vi "Write DetailedResult.vi"(8 "error in (no error)":errorcluster, 10 "DetailedResult":T1, 11 "LocalReport in":refnum<class "LocalReport.lvclass">) -> (0 "error out":errorcluster, 3 "LocalReport out":refnum<class "LocalReport.lvclass">)   [LabVIEW 2019, in "LocalReport.lvlib" / "LocalReport.lvclass"]
uses:
  LocalReport.lvclass
  LocalReport.lvclass/LocalReport.ctl
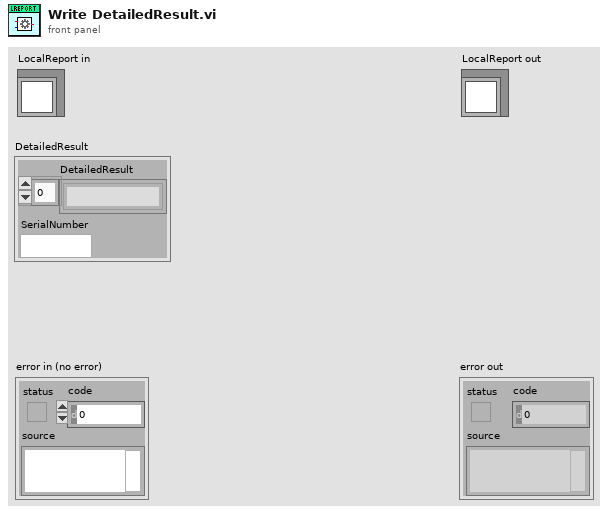
[diagram p1: front panel]
types:
  T1 = cluster{"DetailedResult":string[], "SerialNumber":string}
  T2 = cluster{"TestResultData":string[][], "SerialNumber":string}
  T3 = cluster{"TestResultData":string[][], "SerialNumber":string}[]
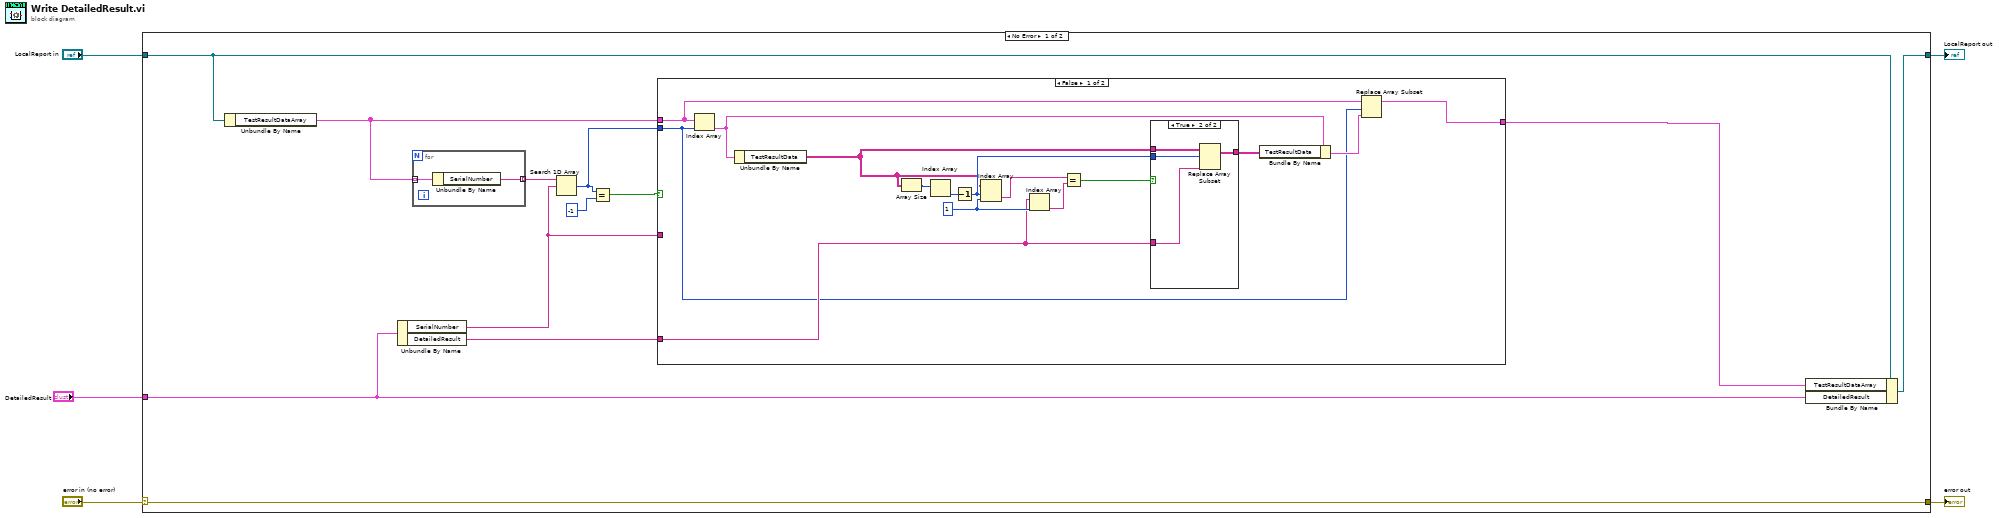
[diagram p0: block diagram]
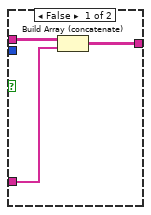
[diagram p2: hidden frame]
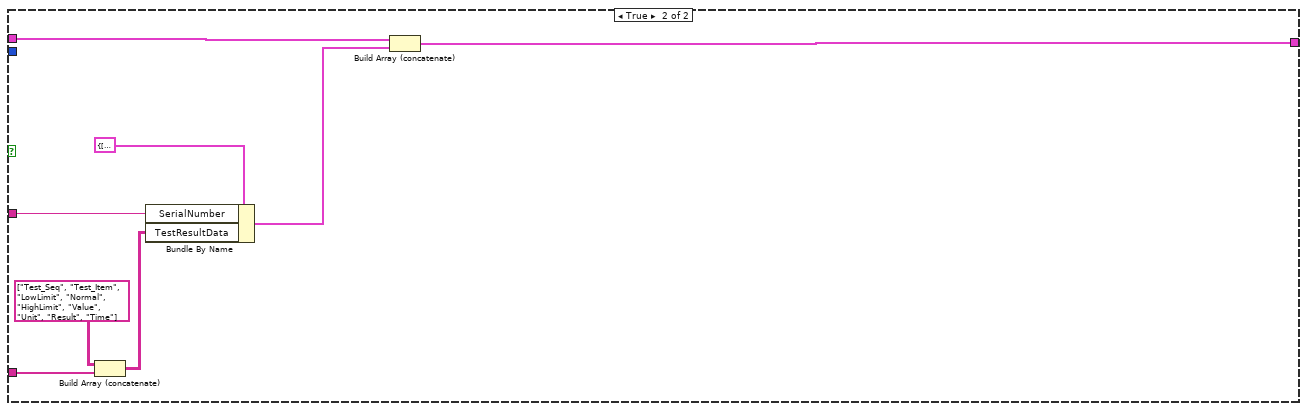
[diagram p3: hidden frame]
diagram:
  n1 = case shown="No Error" "error in (no error)" {
    selector: "error in (no error)" -> [w17 w50]
    tunnel: [w17 w50] -> w4
    tunnel: [w16 w51] -> w2
    tunnel: "LocalReport in" -> [w15 w51]
    tunnel: "DetailedResult" -> [w13 _]
    frame No Error {
      n2 = Unbundle By Name(w15) -> ("TestResultDataArray"=w10:T3)
      n3 = Unbundle By Name(w13) -> ("SerialNumber"=w9:string, "DetailedResult"=w8:string[])
      n4 = for {
        tunnel: w10 -> [w49] mode=indexing
        tunnel: [w48] -> w14 mode=indexing
        n5 = Unbundle By Name(w49) -> ("SerialNumber"=w48:string)
      }
      n6 = Search 1D Array(1D array=w14, element=w9) -> (index of element=w7:i32)  [unwired: 1 in]
      n7 = Equal?(x=w7, y=-1) -> (x = y?=w11:bool)
      n8 = case shown="False" w11 {
        tunnel: w10 -> [w32 w47]
        tunnel: w9 -> [_ w46]
        tunnel: w8 -> [w22 w45]
        tunnel: [w31 w42] -> w6
        tunnel: w7 -> [w18 _]
        frame False {
          w24 = 1 ("禁用的索引 (列)")
          n9 = Index Array(array=w32, index=w18) -> (element=w21:T2)
          n10 = Unbundle By Name(w21) -> ("TestResultData"=w23:string[][])
          n11 = Array Size(array=w23) -> (size(s)=w25:i32[])
          n12 = Index Array(array=w25) -> (element=w26:i32)  [unwired: 1 in]
          n13 = Decrement(x=w26) -> (x-1=w29:i32)
          n14 = Index Array(array=w23, index (row)=w29, index (col)=w24) -> (element=w27:string)
          n15 = Index Array(array=w22, index=w24) -> (element=w28:string)
          n16 = Equal?(x=w27, y=w28) -> (x = y?=w30:bool)
          n17 = case shown="True" w30 {
            tunnel: [w35 w38] -> w20
            tunnel: w23 -> [w34 w39]
            tunnel: w22 -> [w33 w37]
            tunnel: w29 -> [_ w36]
            frame False {
              n18 = Build Array (concatenate)(w34, w33) -> (w35:string[][])
            }
            frame True {
              n19 = Replace Array Subset(array=w39, new element=w37, index (row)=w36) -> (w38:string[][])  [unwired: 1 in]
            }
          }
          n20 = Bundle By Name(cluster=w21, "TestResultData"=w20) -> (w19:T2)
          n21 = Replace Array Subset(array=w32, new element=w19, index=w18) -> (w31:T3)
        }
        frame True {
          n22 = Build Array (concatenate)(string[][] [["Test_Seq", "Test_Item", "LowLimit", "Normal", "HighLimit", "Value", "Unit", "Result", "Time"]] ("TestResultData"), w45) -> (w44:string[][])
          n23 = Bundle By Name(cluster=T2 {"TestResultData"=[["Test_Seq", "Test_Item", "LowLimit", "HighLimit", "Value", "Unit", "Result", "Time"]], "SerialNumber"=""} ("TestResultData"), "SerialNumber"=w46, "TestResultData"=w44) -> (w43:T2)
          n24 = Build Array (concatenate)(w47, w43) -> (w42:T3)
        }
      }
      n25 = Bundle By Name(cluster=w15, "TestResultDataArray"=w6, "DetailedResult"=w13) -> (w16:refnum<class "LocalReport.lvclass">)
    }
    frame Error {
    }
  }
  "error out" <- w4
  "LocalReport out" <- w2
